vi "milan_sketchtosketch.vi"() -> ()   [LabVIEW 2019]
uses:
  <userlib>/IoT Devices/_subVIs/HTTPComm.ctl
  <userlib>/Onshape/_SubVI/Cluster.ctl
  <userlib>/Onshape/_SubVI/z did wid and eid.vi
  <vilib>/picture/picture.llb/Draw True-Color Pixmap.vi
  <userlib>/OnshapeFeatureFunctions/Onshape Feature Funcrions/_SubVI/FS Sketch Polyline.vi
  <userlib>/OnshapeFeatureFunctions/Onshape Feature Funcrions/_SubVI/FS Operation Extrude.vi
panel:
  in  "Scale":i32=50
  in  "file (use dialog)":path
  out "new picture":picture
  out "Numeric":i32
  out "error out":errorcluster
  out "Mouse Modifiers.Button Down":bool
  in  "path to JPEG file":path=path "/Users/milandahal/Desktop/IMG_4335 2.JPG"
  in  "Zoom Factor":sgl(slide) scale=0.1..1.0
  out "Device Out":T1
  out "Comm":T2
  in  "canvas":picture
  in  "stop":bool
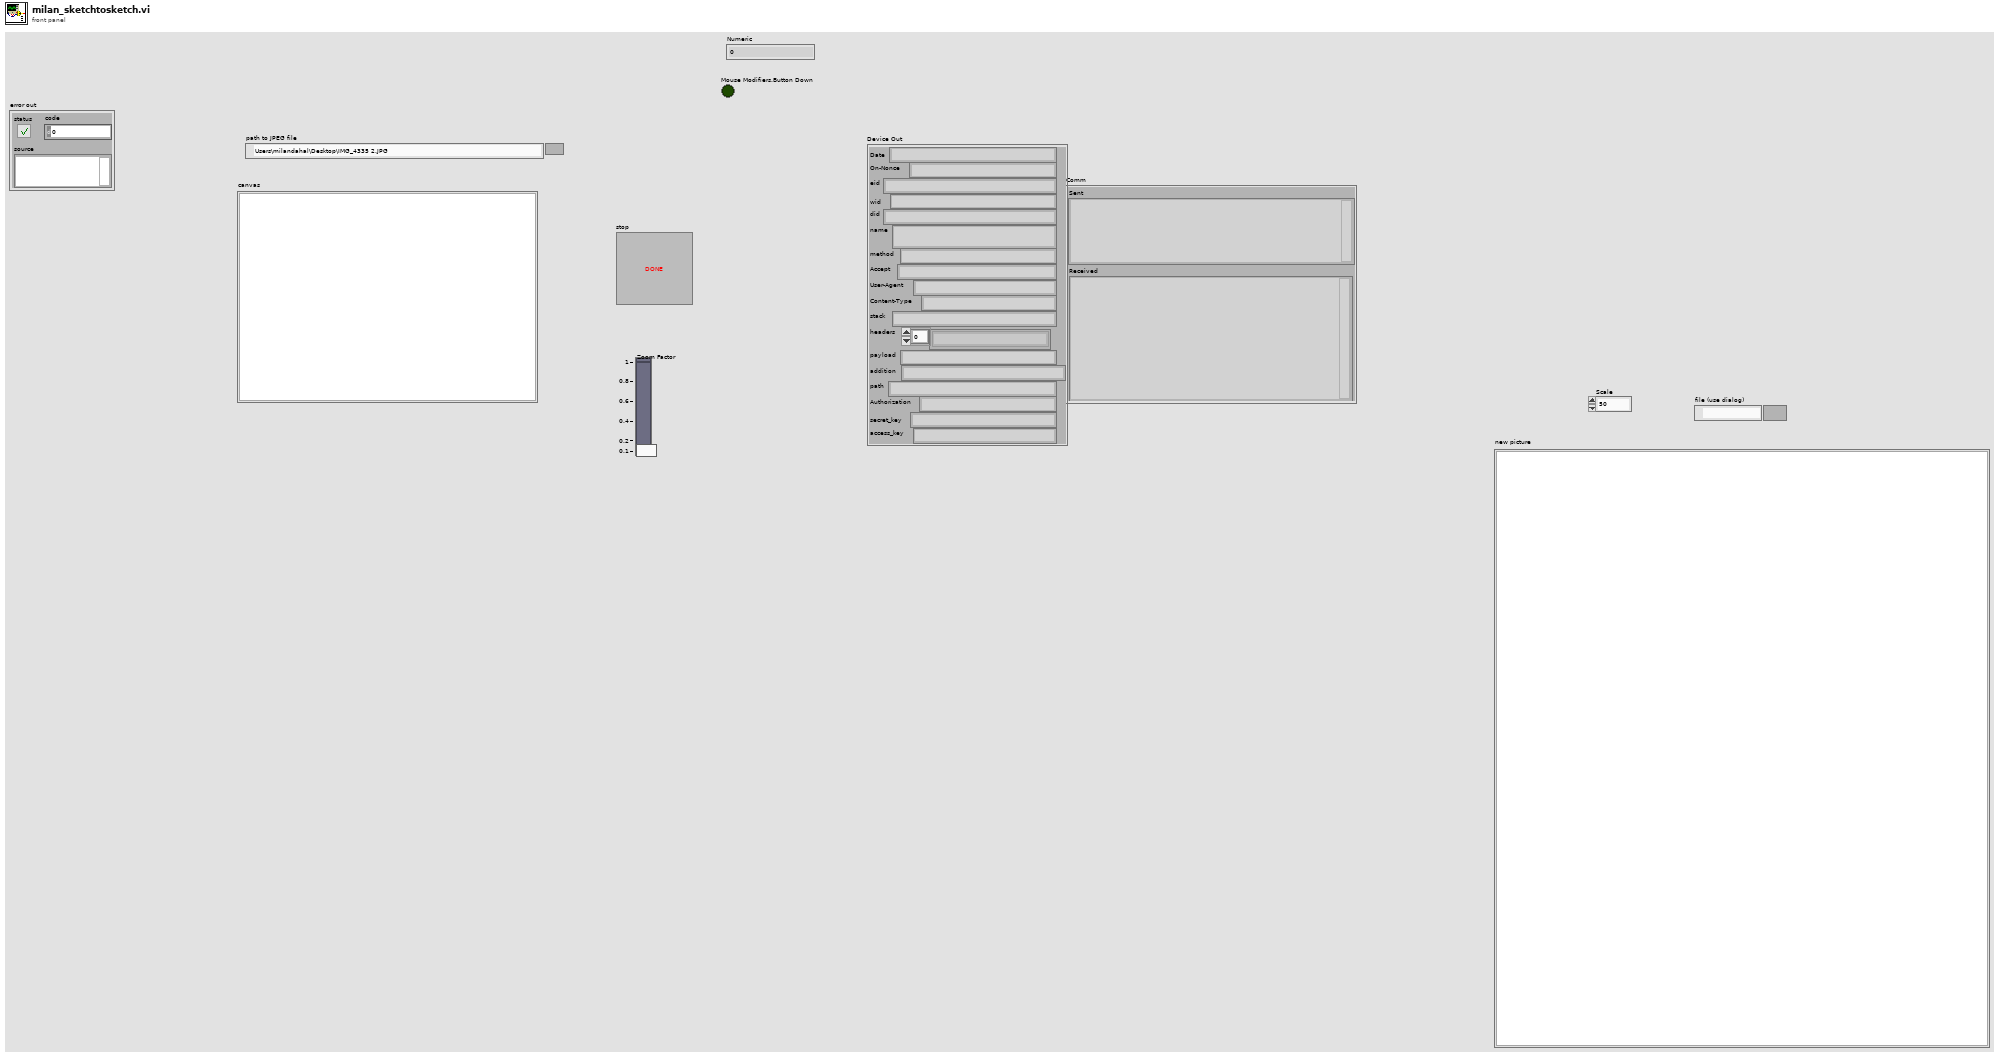
[diagram p1: front panel]
types:
  T1 = typedef "Cluster.ctl" = cluster{"Date":string, "On-Nonce":string, "eid":string, "wid":string, "did":string, "name":string, "method":string, "Accept":string, "User-Agent":string, "Content-Type":string, "stack":string, "headers":string[], "payload":string, "addition":string, "path":string, "Authorization":string, "secret_key":string, "access_key":string}
  T2 = typedef "HTTPComm.ctl" = cluster{"url":string, "sent headers":string, "sent body":string, "headers":string, "body":string, "Sent":string, "Received":string}
  T3 = typedef "imagedata.ctl" = cluster{"image type":i32, "image depth":i32, "image":u8[], "mask":u8[], "colors":u32[], "Rectangle":cluster{"left":i16, "top":i16, "right":i16, "bottom":i16}}
  T4 = typedef "LVMouseTypeDef.ctl" = cluster{"Mouse Position":cluster{"X":i32, "Y":i32}, "Mouse Modifiers":cluster{"Button Down":bool, "Shift Mod":bool, "Menu Mod":bool, "Option Mod":bool}}
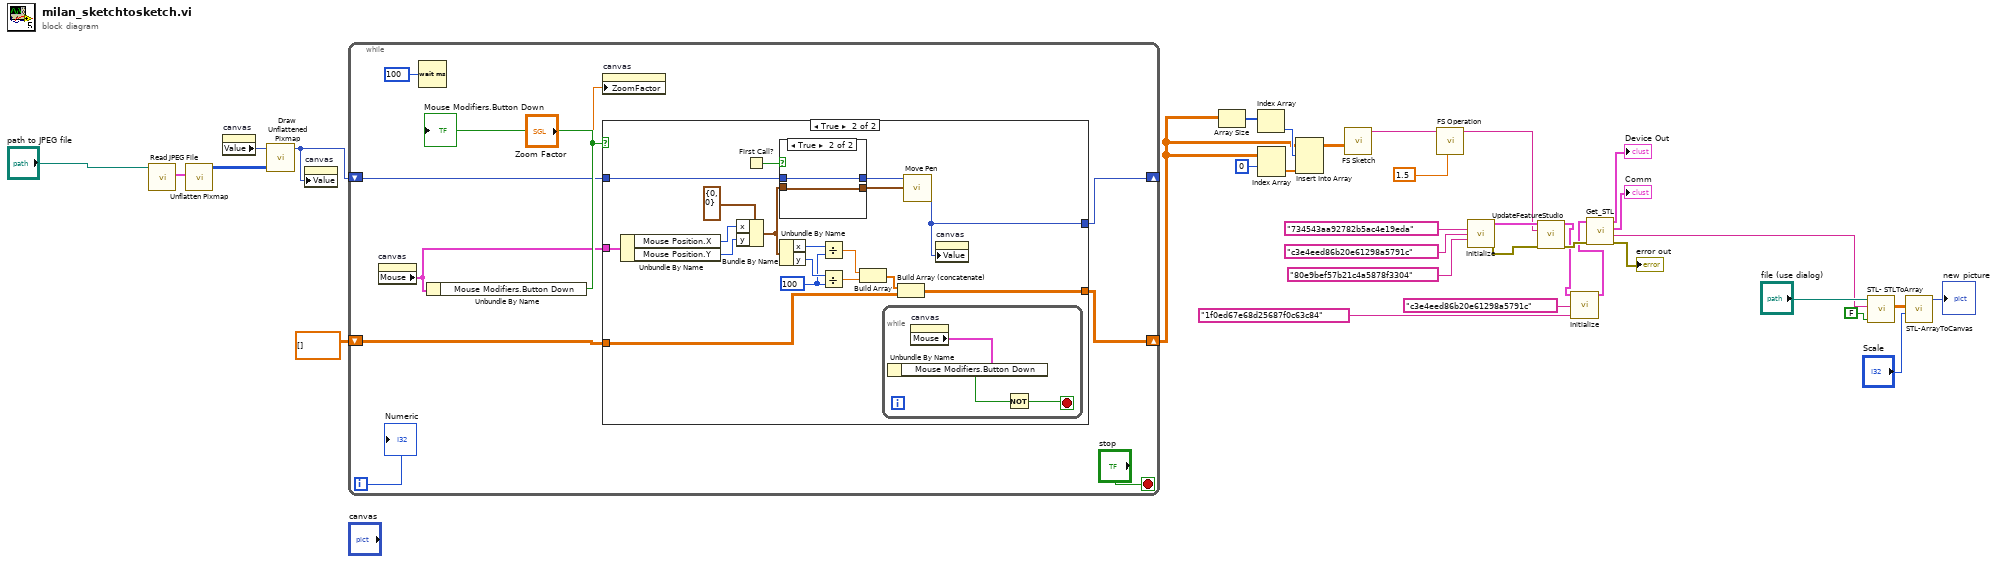
[diagram p0: block diagram]
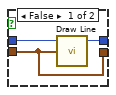
[diagram p3: hidden frame]
diagram:
  n1 = call <vilib>:"Read JPEG File.vi"("path to JPEG file"="path to JPEG file") -> ("image data"=w28:T3)  [unwired: 8 in, 2 out]
  n2 = call <vilib>:"Unflatten Pixmap.vi"("image data"=w28) -> ("24-bit pixmap"=w27:u32[][])  [unwired: 4 in, 6 out]
  n3 = property on="canvas" class="Pict"() -> ("Value"=w29:picture)  [unwired: 2 in, 2 out]
  n4 = call-poly <vilib>:"Draw Unflattened Pixmap.vi"("picture"=w29, "data (RGB format)"=w27) -> ("new picture"=w25:picture)  [unwired: 7 in]
  n5 = property on="canvas" class="Pict"("Value"=w25) -> ()  [unwired: 2 in, 2 out]
  n6 = while {
    shift-right: [w36] -> _
    shift-left: w25 -> [w41]
    shift-right: [w38] -> w18
    shift-left: dbl[][] [] -> [w39]
    i -> [w35]
    stop <- "stop" stop-if-true
    n7 = property on="canvas" class="Pict"() -> ("Mouse"=w40:T4)  [unwired: 2 in, 2 out]
    n8 = Wait (ms)(milliseconds to wait=u32 100) -> ()  [unwired: 1 out]
    n9 = Unbundle By Name(w40) -> ("Mouse Modifiers.Button Down"=w44:bool)
    "Mouse Modifiers.Button Down" <- w44
    n10 = property on="canvas" class="Pict"("ZoomFactor"="Zoom Factor") -> ()  [unwired: 2 in, 2 out]
    n11 = case shown="True" w44 {
      tunnel: w40 -> [_ w61]
      tunnel: w41 -> [w45 w52]
      tunnel: w39 -> [w46 w47]
      tunnel: [w46 w54] -> w38
      tunnel: [w45 w50] -> w36
      frame False {
      }
      frame True {
        w58 = i16 100 ("y")
        n12 = Unbundle By Name(w61) -> ("Mouse Position.X"=w63:i32, "Mouse Position.Y"=w64:i32)
        n13 = Bundle By Name(cluster=cluster{"x":i16, "y":i16} {"x"=0, "y"=0} ("end point"), "x"=w63, "y"=w64) -> (w49:cluster{"x":i16, "y":i16})
        n14 = First Call?() -> (First Call?: T/F=w53:bool)
        n15 = case shown="True" w53 {
          tunnel: w52 -> [w70 w72]
          tunnel: [w69 w72] -> w51
          tunnel: w49 -> [w68 w71]
          tunnel: [w68 w71] -> w48
          frame False {
            n16 = call <vilib>:"Draw Line.vi"("picture"=w70, "end point"=w68) -> ("new picture"=w69:picture)  [unwired: 7 in]
          }
          frame True {
          }
        }
        n17 = Unbundle By Name(w49) -> ("x"=w60:i16, "y"=w59:i16)
        n18 = Divide(x=w60, y=w58) -> (x/y=w57:dbl)
        n19 = Divide(x=w59, y=w58) -> (x/y=w56:dbl)
        n20 = Build Array(w57, w56) -> (w55:dbl[])
        n21 = while {
          stop <- w65 stop-if-true
          n22 = property on="canvas" class="Pict"() -> ("Mouse"=w67:T4)  [unwired: 2 in, 2 out]
          n23 = Unbundle By Name(w67) -> ("Mouse Modifiers.Button Down"=w66:bool)
          n24 = Not(x=w66) -> (.not. x?=w65:bool)
        }
        n25 = Build Array (concatenate)(w55, w47) -> (w54:dbl[][])
        n26 = call <vilib>:"Move Pen.vi"("new position"=w48, "picture"=w51) -> ("new picture"=w50:picture)  [unwired: 3 in]
        n27 = property on="canvas" class="Pict"("Value"=w50) -> ()  [unwired: 2 in, 2 out]
      }
    }
    "Numeric" <- w35
  }
  n28 = Array Size(array=w18) -> (size(s)=w17:i32[])
  n29 = Index Array(array=w17) -> (element=w22:i32)  [unwired: 1 in]
  n30 = Index Array(array=w18, index (row)=0) -> (element=w23:dbl[])  [unwired: 1 in]
  n31 = Insert Into Array(array=w18, index (row)=w22, new element=w23) -> (w8:dbl[][])  [unwired: 1 in]
  n32 = call-poly <userlib>:"FS Sketch.vi"("Polyline Points"=w8) -> ("Feature Out"=w7:string)  [unwired: 10 in]
  n33 = call-poly <userlib>:"FS Operation.vi"("Extrude #"=1.5 ("Extrude Depth"), "Feature In"=w7) -> ("Feature Out"=w20:string)  [unwired: 9 in]
  n34 = call-poly <userlib>:"Initialize.vi"("did"="734543aa92782b5ac4e19eda", "wid"="c3e4eed86b20e61298a5791c", "eid"="80e9bef57b21c4a5878f3304") -> ("Device Out"=w34:T1, "error out"=w30:errorcluster)  [unwired: 11 in]
  n35 = call <userlib>:"UpdateFeatureStudio.vi"("Device In"=w34, "FeatureScript"=w20, "error in"=w30) -> ("Device Out"=w12:T1, "error out"=w14:errorcluster)  [unwired: 10 in, 1 out]
  n36 = call-poly <userlib>:"Initialize.vi"("Device In"=w12, "wid"="c3e4eed86b20e61298a5791c", "eid"="1f0ed67e68d25687f0c63c84") -> ("Device Out"=w11:T1)  [unwired: 11 in, 1 out]
  n37 = call <userlib>:"Get_STL.vi"("error in"=w14, "Device In"=w11) -> ("error out"=→"error out":errorcluster, "stl text"=w1:string, "Comm"=→"Comm":T2, "Device Out"=→"Device Out":T1)  [unwired: 6 in]
  n38 = call "STL- STLToArray.vi"("Boolean"=FALSE, "String"=w1, "file (use dialog)"="file (use dialog)") -> ("Array 3"=w3:dbl[][])  [unwired: 8 in]
  n39 = call "STL-ArrayToCanvas.vi"("Scale"="Scale", "Array 3"=w3) -> ("new picture 3"=→"new picture":picture)  [unwired: 9 in]
